vi "Station_2_ReadInfo.vi"() -> ()   [LabVIEW 2011]
uses:
  <vilib>/Utility/file.llb/Read From Spreadsheet File (string).vi
panel:
  out "Quantity Price":string[](array[string])
  out "Total":string
  out "Quantity":dbl[](array[numeric])
  out "Unit Price":string[](array[string])
  out "Item":string[](array[string])
  out "Price Checker":string
  out "All Items":string[](array[string])
  out "All Prices":string[](array[string])
  out "Euro":dbl
  in  "Amount":dbl
  in  "Currency":string(combo)
  out "Items Folder":string
  out "Match Information":string[][](table)
  out "Colour":u32[][](array[colorbox])
  out "Name and Quantity":string[][](array[string])
  out "ID Image":T1(plugin-control)
  in  "ID Number":string
  in  "Full Program Stop":bool
  in  "Enter ID Number":bool
  out "Method":string
  # "Kevin Mulkearn\n11124725\nUniversity of Limerick"
  # "Instructions:\n1. Run VI.\n2. Insert ID Number.\n3. Insert Currency Amount..\n4. Press 'Enter ID Number' Button.\n5. Press 'STOP' Button to end."
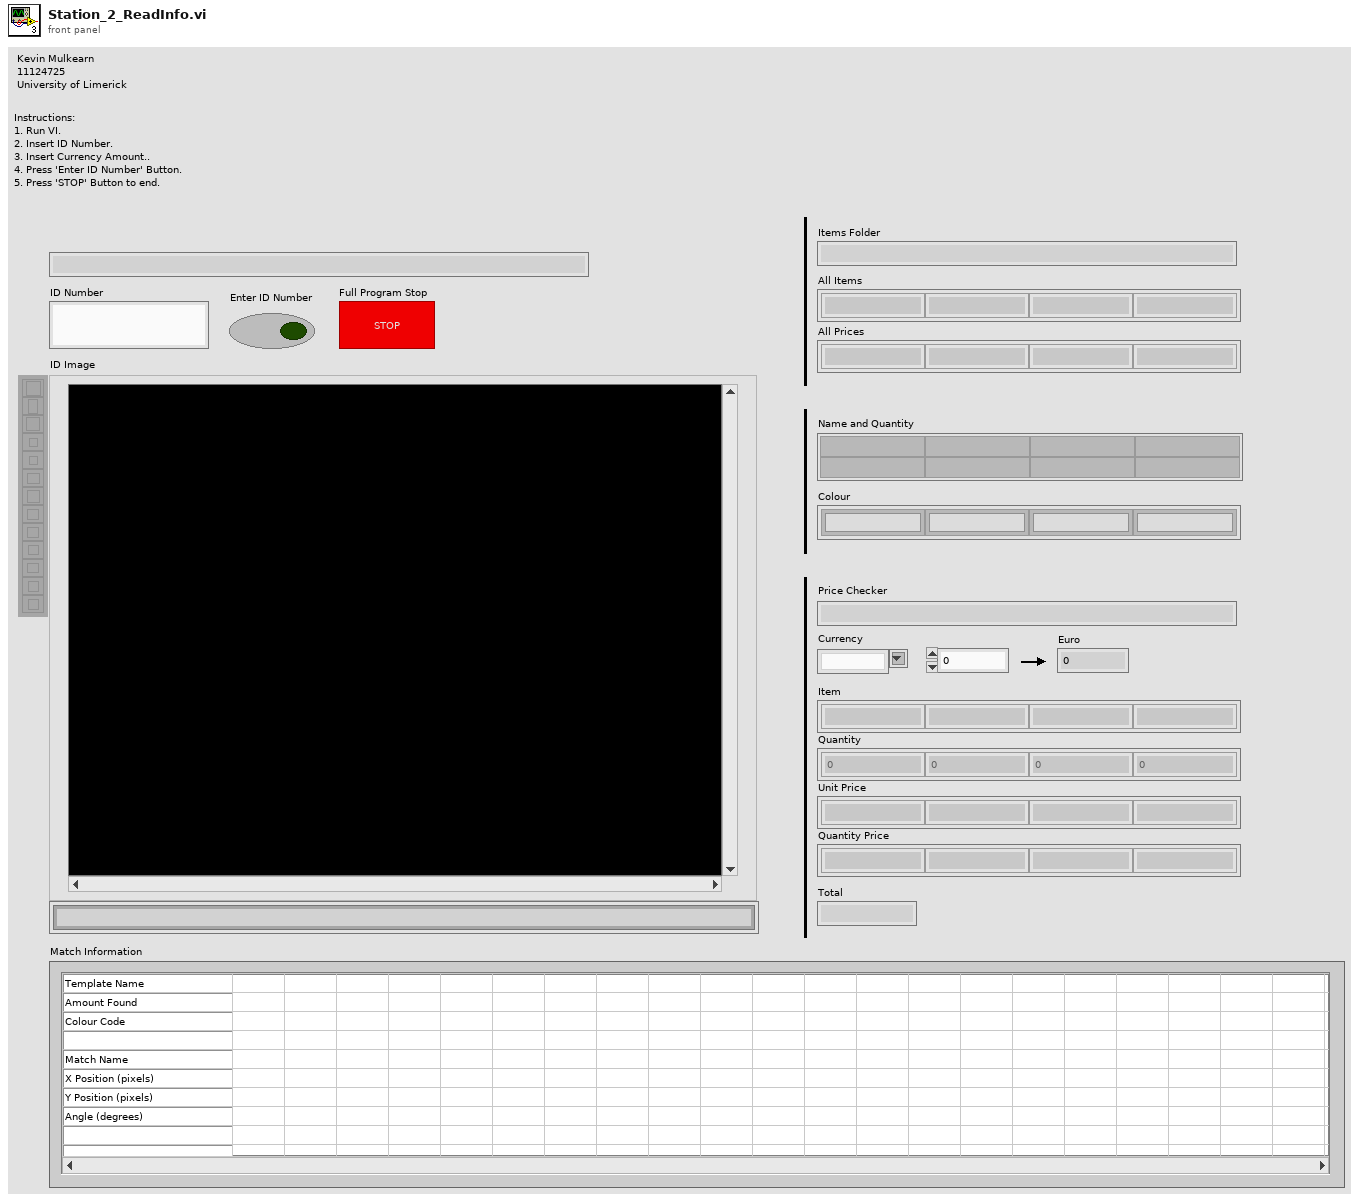
[diagram p1: front panel]
types:
  T1 = typedef "IMAQ Image.ctl" = refnum<image>
  T2 = enum8{"Enabled", "Disabled", "Disabled and Grayed Out"}
  T3 = typedef "Image Type" = u32
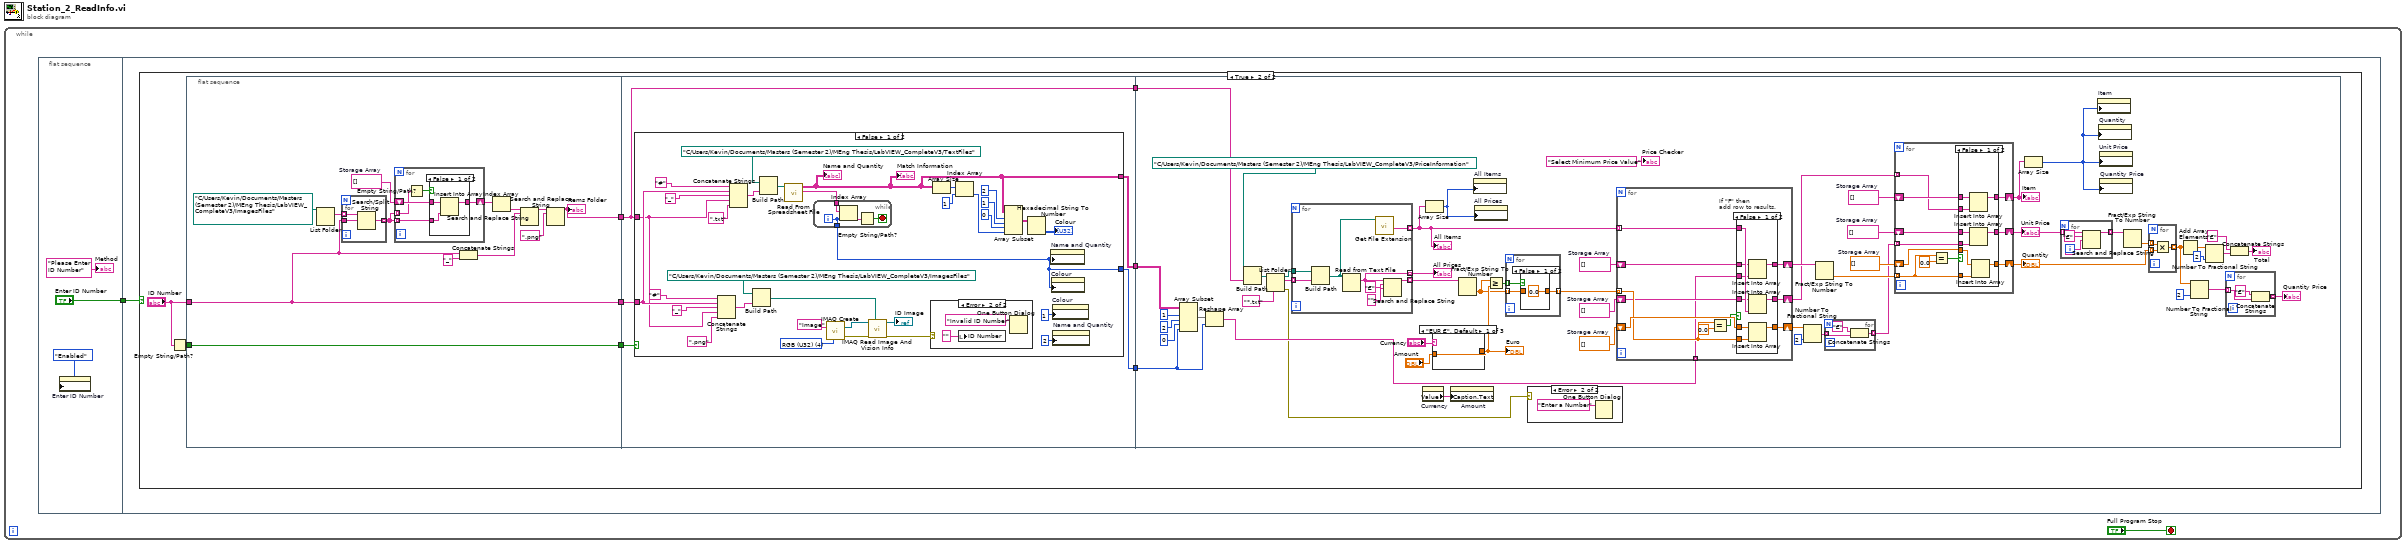
[diagram p0: block diagram]
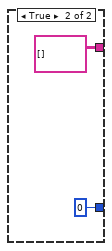
[diagram p5: hidden frame]
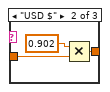
[diagram p10: hidden frame]
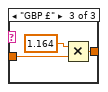
[diagram p11: hidden frame]
diagram:
  n1 = while {
    stop <- "Full Program Stop" stop-if-true
    n2 = flat-sequence {
      tunnel: ["Enter ID Number"] -> w2
      tunnel: w2 -> [w6]
      frame #0 {
        n3 = property on="Enter ID Number" class="Bool"("DisabledEnum"=T2."Enabled" ("Disabled")) -> ()  [unwired: 2 in, 2 out]
        "Method" <- "Please Enter ID Number" ("ID Number 2")
      }
      frame #1 {
        n4 = case shown="True" w6 {
          frame False {
          }
          frame True {
            n5 = Empty String/Path?(string/path="ID Number") -> (empty?=w14:bool)
            n6 = flat-sequence {
              tunnel: "ID Number" -> [w16]
              tunnel: w14 -> [w27]
              tunnel: [w27] -> w12
              tunnel: [w16] -> w11
              tunnel: [w15] -> w10
              tunnel: w12 -> [w44]
              tunnel: w11 -> [w43]
              tunnel: w10 -> [w42]
              tunnel: [w42] -> w9
              tunnel: [w41] -> w8
              tunnel: [w40] -> w7
              tunnel: w9 -> [w139]
              tunnel: w8 -> [w114]
              tunnel: w7 -> [w112]
              frame #0 {
                w20 = string[] []  # Storage Array
                n7 = List Folder(path=path "C:/Users/Kevin/Documents/Masters (Semester 2)/MEng Thesis/LabVIEW_CompleteV3/ImagesFiles" ("Saved Image Location")) -> (filenames=w18:string[])  [unwired: 3 in, 3 out]
                n8 = for {
                  tunnel: w18 -> [w39] mode=indexing
                  tunnel: w16 -> [w38]
                  tunnel: [w37] -> w19 mode=indexing
                  n9 = Search/Split String(string=w39, search string/char (-)=w38) -> (match + rest of string=w37:string)  [unwired: 1 in, 2 out]
                }
                n10 = for {
                  tunnel: w19 -> [w29] mode=indexing
                  tunnel: w19 -> [w30] mode=indexing
                  shift-right: [w32] -> w21
                  shift-left: w20 -> [w31]
                  n11 = Empty String/Path?(string/path=w29) -> (empty?=w28:bool)
                  n12 = case "If \"F\" then \nadd row to results." shown="False" w28 {
                    tunnel: [w35 w36] -> w32
                    tunnel: w31 -> [w34 w36]
                    tunnel: w30 -> [w33 _]
                    frame False {
                      n13 = Insert Into Array(array=w34, new element=w33) -> (w35:string[])  [unwired: 1 in]
                    }
                    frame True {
                    }
                  }
                }
                n14 = Concatenate Strings(w16, "_" ("Image Name")) -> (w24:string)
                n15 = Index Array(array=w21) -> (element=w22:string)  [unwired: 1 in]
                n16 = Search and Replace String(input string=w22, search string=w24) -> (result string=w25:string)  [unwired: 6 in, 3 out]
                n17 = Search and Replace String(input string=w25, search string=".png" ("Image Name")) -> (result string=w15:string)  [unwired: 6 in, 3 out]
                "Items Folder" <- w15
              }
              frame #1 {
                n18 = case shown="False" w44 {
                  tunnel: w43 -> [w66 _]
                  tunnel: w42 -> [w47 _]
                  tunnel: [w46 string[][] [] ("all rows")] -> w41
                  tunnel: [w45 0] -> w40
                  frame False {
                    w70 = T3 4 items=["Grayscale (U8)", "Grayscale (I16)", "Grayscale (SGL)", "Complex (CSG)", "RGB (U32)", "HSL (U32)", "RGB (U64)", "Grayscale (U16)"] ("Image Type")
                    n19 = Concatenate Strings("#" ("string"), w66, "_" ("string"), w47, ".png" ("string")) -> (w75:string)
                    n20 = Concatenate Strings("#" ("string"), w66, "_" ("string"), w47, ".txt" ("string")) -> (w67:string)
                    n21 = Build Path(base path=path "C:/Users/Kevin/Documents/Masters (Semester 2)/MEng Thesis/LabVIEW_CompleteV3/ImagesFiles" ("Saved Image Location"), name or relative path=w75) -> (appended path=w73:path)
                    n22 = Build Path(base path=path "C:/Users/Kevin/Documents/Masters (Semester 2)/MEng Thesis/LabVIEW_CompleteV3/TextFiles" ("Saved Image Location"), name or relative path=w67) -> (appended path=w58:path)
                    n23 = call-poly <vilib>:"Read From Spreadsheet File.vi"("file path (dialog if empty)"=w58) -> ("first row"=w55:string[], "all rows"=w46:string[][])  [unwired: 6 in, 3 out]
                    "Name and Quantity" <- w46
                    "Match Information" <- w46
                    n24 = while {
                      tunnel: w55 -> [w82]
                      tunnel: [w80] -> w45
                      i -> [w80]
                      stop <- w81 stop-if-true
                      n25 = Index Array(array=w82, index=w80) -> (element=w83:string)
                      n26 = Empty String/Path?(string/path=w83) -> (empty?=w81:bool)
                    }
                    n27 = call "IMAQ Create"("Image Name"="Image", "Image Type"=w70) -> ("New Image"=w74:T1, "error out"=w53:errorcluster)  [unwired: 2 in, 1 out]
                    n28 = call "IMAQ Read Image And Vision Info"("File Path"=w73, "error in (no error)"=w53, "Image"=w74) -> ("error out"=w52:errorcluster, "Image Out"=→"ID Image":T1)  [unwired: 1 in, 6 out]
                    n29 = case shown="Error" w52 {
                      frame No Error {
                      }
                      frame Error {
                        n30 = local write "ID Number"("" ("ID Number 2")) -> ()
                        n31 = One Button Dialog(message="Invalid ID Number") -> ()  [unwired: 1 in, 1 out]
                      }
                    }
                    n32 = Array Size(array=w46) -> (size(s)=w61:i32[])
                    n33 = Index Array(array=w61, index=1) -> (element=w59:i32)
                    n34 = Array Subset(array=w46, index (row)=2 ("index"), length (row)=1 ("length"), index (col)=0 ("index 2"), length (col)=w59) -> (w56:string[][])
                    n35 = Hexadecimal String To Number(string=w56) -> (number=→"Colour":u32[][])  [unwired: 2 in, 1 out]
                    n36 = property on="Name and Quantity" class="Arr (strict)"("Number of Columns"=w45) -> ()  [unwired: 2 in, 2 out]
                    n37 = property on="Colour" class="Arr (strict)"("Number of Columns"=w45) -> ()  [unwired: 2 in, 2 out]
                    n38 = property on="Colour" class="Arr (strict)"("Number of Rows"=u32 1) -> ()  [unwired: 2 in, 2 out]
                    n39 = property on="Name and Quantity" class="Arr (strict)"("Number of Rows"=u32 2) -> ()  [unwired: 2 in, 2 out]
                  }
                  frame True {
                  }
                }
              }
              frame #2 {
                w104 = string[] []  # Storage Array
                w103 = string[] []  # Storage Array
                w106 = dbl[] []  # Storage Array
                w110 = string[] []  # Storage Array
                w125 = string[] []  # Storage Array
                w128 = dbl[] []  # Storage Array
                n40 = Array Subset(array=w114, index (row)=1 ("index"), length (row)=2 ("length"), index (col)=0 ("index 2"), length (col)=w112) -> (w113:string[][])
                n41 = Reshape Array(w113, w112) -> (w111:string[])
                n42 = Build Path(base path=path "C:/Users/Kevin/Documents/Masters (Semester 2)/MEng Thesis/LabVIEW_CompleteV3/PriceInformation" ("Price Location"), name or relative path=w139) -> (appended path=w120:path)
                n43 = List Folder(path=w120, pattern="*.txt") -> (path out=w134:path, filenames=w133:string[], error out=w108:errorcluster)  [unwired: 2 in, 1 out]
                n44 = for {
                  tunnel: [w210] -> w129 mode=indexing
                  tunnel: w134 -> [w209]
                  tunnel: w133 -> [w208] mode=indexing
                  tunnel: [w207] -> w132 mode=indexing
                  tunnel: [w205] -> w124 mode=indexing
                  n45 = Build Path(base path=w209, name or relative path=w208) -> (appended path=w206:path)
                  n46 = Read from Text File(file (use dialog)=w206) -> (text=w207:string)  [unwired: 3 in, 3 out]
                  n47 = call <vilib>:"Get File Extension.vi"("file"=w206) -> ("filename without extension"=w205:string)  [unwired: 7 in, 3 out]
                  n48 = Search and Replace String(input string=w207, search string="€", replace string="" ("replace string (\"\")")) -> (result string=w210:string)  [unwired: 5 in, 3 out]
                }
                "All Prices" <- w132
                "All Items" <- w124
                n49 = property on="Currency" class="CmbBox"() -> ("Value"=w136:string)  [unwired: 2 in, 2 out]
                n50 = Array Size(array=w124) -> (size(s)=w107:i32)
                n51 = case shown="\"EUR €\", Default" "Currency" {
                  tunnel: "Amount" -> [w213 w216 w219]
                  tunnel: [w213 w215 w218] -> w131
                  frame "EUR €", Default {
                  }
                  frame "USD $" {
                    n52 = Multiply(x=0.902, y=w216) -> (x*y=w215:dbl)
                  }
                  frame "GBP £" {
                    n53 = Multiply(x=1.164, y=w219) -> (x*y=w218:dbl)
                  }
                }
                "Euro" <- w131
                n54 = property on="Amount" class="DigNum (strict)"("Caption.Text"=w136) -> ()  [unwired: 2 in, 2 out]
                n55 = Fract/Exp String To Number(string=w129) -> (number=w126:dbl[])  [unwired: 3 in, 1 out]
                n56 = property on="All Items" class="Arr (strict)"("Number of Columns"=w107) -> ()  [unwired: 2 in, 2 out]
                n57 = property on="All Prices" class="Arr (strict)"("Number of Columns"=w107) -> ()  [unwired: 2 in, 2 out]
                n58 = Greater Or Equal?(x=w126, y=w131) -> (x >= y?=w130:bool[])
                n59 = for {
                  tunnel: w130 -> [w202] mode=indexing
                  tunnel: [w201] -> w127 mode=indexing
                  tunnel: w126 -> [w200] mode=indexing
                  n60 = case shown="False" w202 {
                    tunnel: [0.0 ("result string") w204] -> w201
                    tunnel: w200 -> [_ w204]
                    frame False {
                    }
                    frame True {
                    }
                  }
                }
                n61 = case shown="Error" w108 {
                  frame No Error {
                  }
                  frame Error {
                    n62 = One Button Dialog(message="Enter a Number") -> ()  [unwired: 1 in, 1 out]
                  }
                }
                n63 = for {
                  tunnel: w127 -> [w185] mode=indexing
                  shift-right: [w186] -> w119
                  shift-left: w128 -> [w187]
                  tunnel: w124 -> [w181] mode=indexing
                  shift-right: [w182] -> w102
                  shift-left: w125 -> [w180]
                  tunnel: w111 -> [w179] mode=indexing
                  shift-right: [w177] -> w109
                  shift-left: w110 -> [w178]
                  n64 = Equal?(x=w185, y=0.0) -> (x = y?=w183:bool)
                  n65 = case "If \"F\" then \nadd row to results." shown="False" w183 {
                    tunnel: w187 -> [w196 w199]
                    tunnel: w185 -> [w195 _]
                    tunnel: [w194 w199] -> w186
                    tunnel: [w193 w198] -> w182
                    tunnel: w181 -> [w192 _]
                    tunnel: w180 -> [w191 w198]
                    tunnel: w179 -> [w190 _]
                    tunnel: w178 -> [w189 w197]
                    tunnel: [w188 w197] -> w177
                    frame False {
                      n66 = Insert Into Array(array=w189, new element=w190) -> (w188:string[])  [unwired: 1 in]
                      n67 = Insert Into Array(array=w191, new element=w192) -> (w193:string[])  [unwired: 1 in]
                      n68 = Insert Into Array(array=w196, new element=w195) -> (w194:dbl[])  [unwired: 1 in]
                    }
                    frame True {
                    }
                  }
                }
                n69 = Number To Fractional String(number=w119, precision (6)=i16 2) -> (F-format string=w122:string[])  [unwired: 2 in]
                n70 = Fract/Exp String To Number(string=w109) -> (number=w105:dbl[])  [unwired: 3 in, 1 out]
                n71 = for {
                  tunnel: w122 -> [w175] mode=indexing
                  tunnel: [w176] -> w101 mode=indexing
                  n72 = Concatenate Strings("€" ("string"), w175) -> (w176:string)
                }
                n73 = for {
                  shift-right: [w159] -> w97
                  shift-left: w106 -> [w160]
                  shift-right: [w156] -> w100
                  shift-left: w104 -> [w155]
                  shift-right: [w153] -> w87
                  shift-left: w103 -> [w154]
                  tunnel: w105 -> [w152] mode=indexing
                  tunnel: w102 -> [w151] mode=indexing
                  tunnel: w101 -> [w150] mode=indexing
                  n74 = Equal?(x=w152, y=0.0) -> (x = y?=w157:bool)
                  n75 = case "If \"F\" then \nadd row to results." shown="False" w157 {
                    tunnel: w160 -> [w166 w172]
                    tunnel: [w169 w172] -> w159
                    tunnel: [w168 w171] -> w156
                    tunnel: w155 -> [w163 w171]
                    tunnel: w154 -> [w164 w170]
                    tunnel: [w167 w170] -> w153
                    tunnel: w152 -> [w165 _]
                    tunnel: w151 -> [w162 _]
                    tunnel: w150 -> [w161 _]
                    frame False {
                      n76 = Insert Into Array(array=w164, new element=w162) -> (w167:string[])  [unwired: 1 in]
                      n77 = Insert Into Array(array=w163, new element=w161) -> (w168:string[])  [unwired: 1 in]
                      n78 = Insert Into Array(array=w166, new element=w165) -> (w169:dbl[])  [unwired: 1 in]
                    }
                    frame True {
                    }
                  }
                }
                "Item" <- w87
                "Unit Price" <- w100
                "Quantity" <- w97
                n79 = Array Size(array=w87) -> (size(s)=w86:i32)
                n80 = for {
                  tunnel: w100 -> [w147] mode=indexing
                  tunnel: [w146] -> w99 mode=indexing
                  n81 = Search and Replace String(input string=w147, search string="€", replace string="" ("replace string (\"\")")) -> (result string=w146:string)  [unwired: 5 in, 3 out]
                }
                n82 = property on="Item" class="Arr (strict)"("Number of Columns"=w86) -> ()  [unwired: 2 in, 2 out]
                n83 = property on="Quantity" class="Arr (strict)"("Number of Columns"=w86) -> ()  [unwired: 2 in, 2 out]
                n84 = property on="Unit Price" class="Arr (strict)"("Number of Columns"=w86) -> ()  [unwired: 2 in, 2 out]
                n85 = property on="Quantity Price" class="Arr (strict)"("Number of Columns"=w86) -> ()  [unwired: 2 in, 2 out]
                n86 = Fract/Exp String To Number(string=w99) -> (number=w98:dbl[])  [unwired: 3 in, 1 out]
                n87 = for {
                  tunnel: w98 -> [w145] mode=indexing
                  tunnel: w97 -> [w144] mode=indexing
                  tunnel: [w143] -> w90 mode=indexing
                  n88 = Multiply(x=w145, y=w144) -> (x*y=w143:dbl)
                }
                n89 = Add Array Elements(numeric array=w90) -> (sum=w95:dbl)
                n90 = Number To Fractional String(number=w90, precision (6)=i16 2) -> (F-format string=w89:string[])  [unwired: 2 in]
                n91 = Number To Fractional String(number=w95, precision (6)=i16 2) -> (F-format string=w93:string)  [unwired: 2 in]
                n92 = for {
                  tunnel: w89 -> [w141] mode=indexing
                  tunnel: [w142] -> w88 mode=indexing
                  n93 = Concatenate Strings("€" ("string"), w141) -> (w142:string)
                }
                "Quantity Price" <- w88
                n94 = Concatenate Strings("€" ("string"), w93) -> (→"Total":string)
                "Price Checker" <- "Select Minimum Price Value" ("String")
              }
            }
          }
        }
      }
    }
  }
